vi "solar_log Banner.vi"(7 "Close? (F)":bool, 8 "error in (no error)":errorcluster, 10 "Error Summary":string="Unknown Error", 11 "Error Code":i32) -> (0 "error out":errorcluster)   [LabVIEW 2018]
doc: "This launches the error notification bar across the top of the primary monitor."
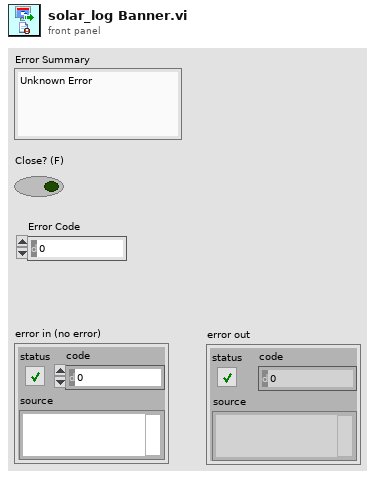
[diagram p1: front panel]
types:
  T1 = enum32{"Invalid", "Standard", "Closed", "Hidden", "Minimized", "Maximized"}
  T2 = enum32{"Bad", "Idle", "Run top level", "Running"}
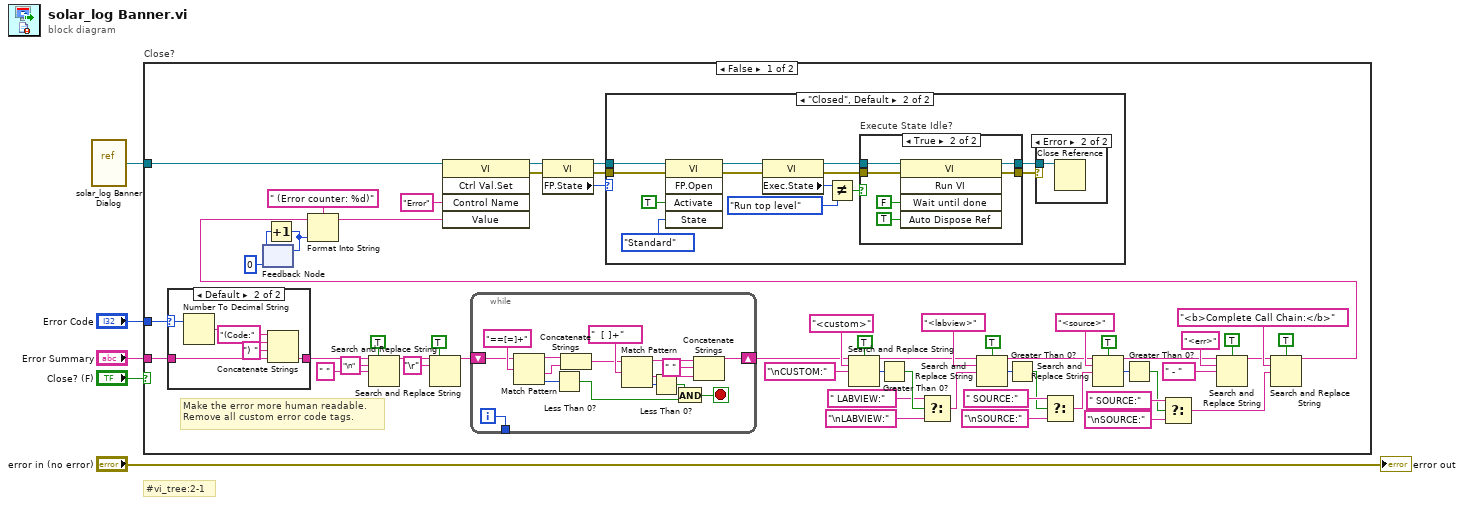
[diagram p0: block diagram]
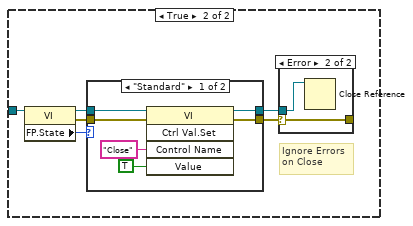
[diagram p6: hidden frame]
diagram:
  # "#vi_tree:2-1"
  n1 = vi-ref "solar_log Banner Dialog.vi"() -> (w4:refnum<vi>)
  n2 = case "Close?" shown="False" "Close? (F)" {
    tunnel: w4 -> [w12 w111]
    tunnel: "Error Summary" -> [w54 _]
    tunnel: "Error Code" -> [w32 _]
    frame False {
      # "Make the error more human readable.\nRemove all custom error code tags."
      n3 = case shown="Default" w32 {
        selector: w32 -> [_ w102]
        tunnel: w54 -> [w99 w105]
        tunnel: [w99 w104] -> w33
        frame 0 {
        }
        frame Default {
          n4 = Number To Decimal String(number=w102) -> (decimal integer string=w103:string)  [unwired: 1 in]
          n5 = Concatenate Strings("(Code:" ("string"), w103, ") " ("string"), w105) -> (w104:string)
        }
      }
      n6 = feedback #1(0) -> (w11:i32)
      n7 = Increment(x=w11) -> (x+1=w9:i32)
      n8 = feedback-in #1(w9) -> ()
      n9 = Search and Replace String(replace all?=TRUE ("ignore case? (F)"), input string=w33, search string="\n", replace string=" " ("replace string (\"\")")) -> (result string=w48:string)  [unwired: 4 in, 3 out]
      n10 = Search and Replace String(replace all?=TRUE ("ignore case? (F)"), input string=w48, search string="\r") -> (result string=w21:string)  [unwired: 5 in, 3 out]
      n11 = while {
        shift-right: [w90] -> w20
        shift-left: w21 -> [w95]
        tunnel: [w84] -> _
        i -> [w84]
        stop <- w85 stop-if-true
        n12 = Match Pattern(string=w95, regular expression="==[=]+") -> (before substring=w97:string, after substring=w96:string, offset past match=w88:i32)  [unwired: 1 in, 1 out]
        n13 = Less Than 0?(x=w88) -> (x < 0?=w86:bool)
        n14 = Concatenate Strings(w97, w96) -> (w91:string)
        n15 = Match Pattern(string=w91, regular expression="  [ ]+") -> (before substring=w93:string, after substring=w94:string, offset past match=w89:i32)  [unwired: 1 in, 1 out]
        n16 = Less Than 0?(x=w89) -> (x < 0?=w87:bool)
        n17 = And(x=w87, y=w86) -> (x .and. y?=w85:bool)
        n18 = Concatenate Strings(w93, " " ("string"), w94) -> (w90:string)
      }
      n19 = Search and Replace String(case sensitive?=TRUE ("ignore case? (F)"), input string=w20, search string="<custom>", replace string="\nCUSTOM:" ("replace string (\"\")")) -> (result string=w42:string, number of replacements=w41:i32)  [unwired: 4 in, 2 out]
      n20 = Greater Than 0?(x=w41) -> (x > 0?=w40:bool)
      n21 = Select(t=" LABVIEW:" ("replace string (\"\")"), s=w40, f="\nLABVIEW:" ("replace string (\"\")")) -> (s? t:f=w37:string)
      n22 = Search and Replace String(case sensitive?=TRUE ("ignore case? (F)"), input string=w42, search string="<labview>", replace string=w37) -> (result string=w19:string, number of replacements=w31:i32)  [unwired: 4 in, 2 out]
      n23 = Greater Than 0?(x=w31) -> (x > 0?=w28:bool)
      n24 = Select(t=" SOURCE:" ("replace string (\"\")"), s=w28, f="\nSOURCE:" ("replace string (\"\")")) -> (s? t:f=w27:string)
      n25 = Search and Replace String(case sensitive?=TRUE ("ignore case? (F)"), input string=w19, search string="<source>", replace string=w27) -> (result string=w34:string, number of replacements=w24:i32)  [unwired: 4 in, 2 out]
      n26 = Greater Than 0?(x=w24) -> (x > 0?=w23:bool)
      n27 = Select(t=" SOURCE:" ("replace string (\"\")"), s=w23, f="\nSOURCE:" ("replace string (\"\")")) -> (s? t:f=w22:string)
      n28 = Search and Replace String(case sensitive?=TRUE ("ignore case? (F)"), input string=w34, search string="<err>", replace string=" - " ("search string")) -> (result string=w55:string)  [unwired: 4 in, 3 out]
      n29 = Search and Replace String(case sensitive?=TRUE ("ignore case? (F)"), input string=w55, search string="<b>Complete Call Chain:</b>", replace string=w22) -> (result string=w6:string)  [unwired: 4 in, 3 out]
      n30 = Format Into String(format string=" (Error counter: %d)", initial string=w6, w9) -> (resulting string=w7:string)  [unwired: 1 in, 1 out]
      n31 = invoke class="VI" method="Ctrl Val.Set"(reference=w12, "Control Name"="Error", "Value"=w7) -> (reference out=w17:refnum<vi>, error out=w16:errorcluster)  [unwired: 2 in, 3 out]
      n32 = property class="VI"(reference=w17, error in=w16) -> (reference out=w14:refnum<vi>, error out=w15:errorcluster, "FP.State"=w13:T1)
      n33 = case shown="\"Closed\", Default" w13 {
        tunnel: w15 -> [_ w63]
        tunnel: w14 -> [_ w61]
        frame "Standard" {
        }
        frame "Closed", Default {
          n34 = invoke class="VI" method="FP.Open"(reference=w61, error in=w63, "Activate"=TRUE ("Activate?"), "State"=T1."Standard") -> (reference out=w66:refnum<vi>, error out=w67:errorcluster)  [unwired: 1 in, 3 out]
          n35 = property on="Property Node" class="VI"(reference=w66, error in=w67) -> (reference out=w72:refnum<vi>, error out=w73:errorcluster, "Exec.State"=w71:T2)
          n36 = Not Equal?(x=w71, y=T2."Run top level" ("Execution:State")) -> (x != y?=w62:bool)
          n37 = case "Execute State Idle?" shown="True" w62 {
            tunnel: w73 -> [w74 w81]
            tunnel: w72 -> [w75 w80]
            tunnel: [w74 w79] -> w69
            tunnel: [w75 w78] -> w68
            frame False {
            }
            frame True {
              n38 = invoke class="VI" method="Run VI"(reference=w80, error in=w81, "Wait until done"=FALSE ("Wait Until Done"), "Auto Dispose Ref"=TRUE ("Auto Dispose Reference")) -> (reference out=w78:refnum<vi>, error out=w79:errorcluster)  [unwired: 1 in, 3 out]
            }
          }
          n39 = case shown="Error" w69 {
            tunnel: w68 -> [_ w82]
            frame No Error {
            }
            frame Error {
              n40 = Close Reference(reference=w82) -> ()  [unwired: 1 in, 1 out]
            }
          }
        }
      }
    }
    frame True {
      # "Ignore Errors on Close"
      n41 = property class="VI"(reference=w111) -> (reference out=w109:refnum<vi>, error out=w110:errorcluster, "FP.State"=w106:T1)  [unwired: 1 in]
      n42 = case shown="\"Standard\"" w106 {
        tunnel: [w115 w118] -> w108
        tunnel: [w114 w119] -> w107
        tunnel: w110 -> [w116 w118]
        tunnel: w109 -> [w117 w119]
        frame "Standard" {
          n43 = invoke class="VI" method="Ctrl Val.Set"(reference=w117, error in=w116, "Control Name"="Close", "Value"=TRUE) -> (reference out=w114:refnum<vi>, error out=w115:errorcluster)  [unwired: 1 in, 3 out]
        }
        frame Default {
        }
      }
      n44 = case shown="Error" w108 {
        selector: w108 -> [w120 w121]
        tunnel: w107 -> [_ w122]
        tunnel: [w120 w121] -> _
        frame No Error {
        }
        frame Error {
          n45 = Close Reference(reference=w122) -> ()  [unwired: 1 in, 1 out]
        }
      }
    }
  }
  "error out" <- "error in (no error)"
